vi "Configure Aperture Timing.vi"(0 "VISA resource name":refnum<visa-resource-name>, 1 "Scan List (Empty)":string, 5 "Timing Units (0: Seconds)":u16(ring) items=["Seconds", "Power Line Cycles"], 7 "Timing Value (0.020)":dbl=0.02, 11 "error in (no error)":errorcluster) -> (4 "VISA resource name out":refnum<visa-resource-name>, 15 "error out":errorcluster)   [LabVIEW 2020, in "Keithley 27XX.lvlib"]
doc: "This VI configures the integration time, or aperture, of the A/D converter for the current measurement function.\n\nNote: \n(1) Configure Measurement.vi must be called <B>before</B> setting the timing.\n\n(2) Frequency: Does not allow NPLC for units\nPeriod: Does not allow NPLC for units\nContinuity: Does not allow for configuration of timing.\n\n(3) This VI should not be run when measurement mode is set to continuity."
uses:
  Keithley 27XX.lvlib
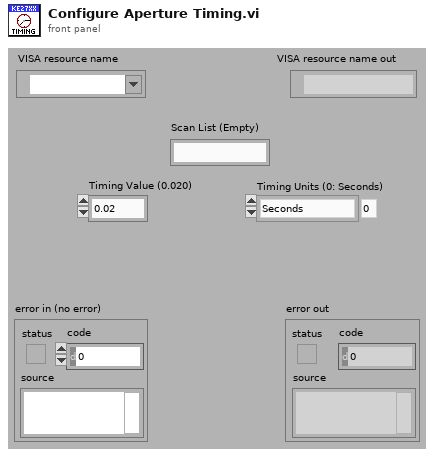
[diagram p1: front panel]
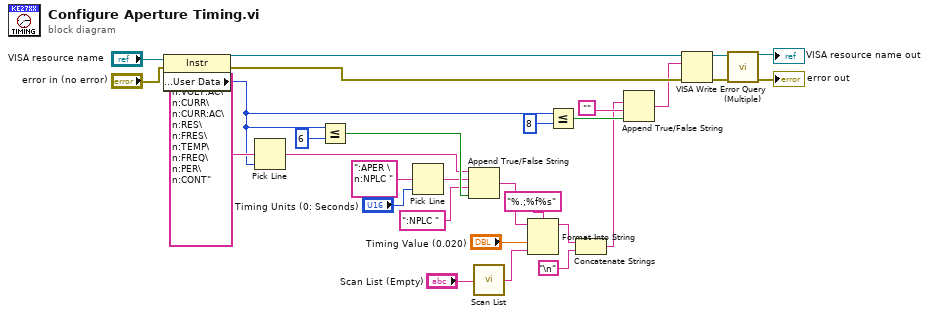
[diagram p0: block diagram]
diagram:
  n1 = property on="Property Node" class="Instr"(reference="VISA resource name", error in="error in (no error)") -> (reference out=w26:refnum<visa-resource-name>, error out=w25:errorcluster, "General Settings:User Data"=w4:u32)
  n2 = Pick Line(multi-line string=":VOLT\n:VOLT:AC\n:CURR\n:CURR:AC\n:RES\n:FRES\n:TEMP\n:FREQ\n:PER\n:CONT", line index=w4) -> (output string=w5:string)  [unwired: 1 in]
  n3 = Less Or Equal?(x=w4, y=6) -> (x <= y?=w10:bool)
  n4 = Pick Line(multi-line string=":APER \n:NPLC ", line index="Timing Units (0: Seconds)") -> (output string=w9:string)  [unwired: 1 in]
  n5 = Append True/False String(1:w10, 2:":NPLC " ("false string"), 3:w9, 4:w5) -> (0:w11:string)
  n6 = call "Scan List.vi"("Scan List (Empty)"="Scan List (Empty)") -> ("Scan List Out"=w20:string)  [unwired: 14 in]
  n7 = Format Into String(format string="%.;%f%s", initial string=w11, "Timing Value (0.020)", w20) -> (resulting string=w2:string)  [unwired: 1 in, 1 out]
  n8 = Less Or Equal?(x=w4, y=8) -> (x <= y?=w6:bool)
  n9 = Concatenate Strings(w2, "\n") -> (w1:string)
  n10 = Append True/False String(1:w6, 2:"", 3:w1) -> (0:w12:string)  [unwired: 1 in]
  n11 = VISA Write(VISA resource name=w26, write buffer=w12, error in (no error)=w25) -> (VISA resource name out=w18:refnum<visa-resource-name>, error out=w17:errorcluster)  [unwired: 1 out]
  n12 = call "Error Query (Multiple).vi"("VISA resource name"=w18, "error in (no error)"=w17) -> ("VISA resource name out"=→"VISA resource name out":refnum<visa-resource-name>, "error out"=→"error out":errorcluster)  [unwired: 10 in, 2 out]
